vi "Get Value.vi"(8 "error in (no error)":errorcluster, 11 "SingleA in":refnum<class "SingleA.lvclass">) -> (0 "error out":errorcluster, 2 "value":dbl, 3 "SingleA out":refnum<class "SingleA.lvclass">)   [LabVIEW 2020, in "SingleA.lvclass"]
uses:
  SingleA.lvclass
  D:/03 GitHub/LabVIEW-Singleton/Singleton/Singleton.lvclass
  Singleton/Singleton.lvclass/Singleton.ctl
  SingleA.lvclass/SingleA.ctl
  Singleton/Singleton.lvclass
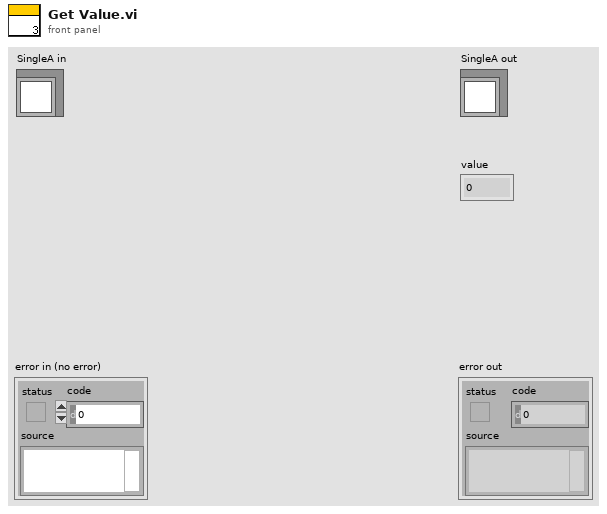
[diagram p1: front panel]
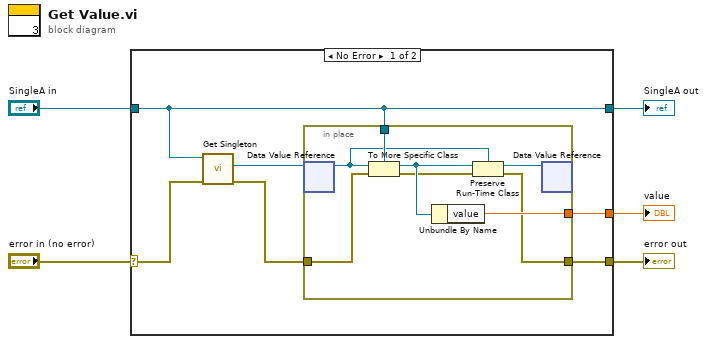
[diagram p0: block diagram]
diagram:
  n1 = case shown="No Error" "error in (no error)" {
    selector: "error in (no error)" -> [w8 w21]
    tunnel: [w7 w21] -> w4
    tunnel: [w10 w20] -> w2
    tunnel: "SingleA in" -> [w10 w20]
    tunnel: [w9 _] -> w1
    frame No Error {
      n2 = call "Get Singleton.vi"("error in (no error)"=w8, "Singleton in"=w10) -> ("error out"=w6:errorcluster, "singleton"=w11:refnum<data-value>)  [unwired: 7 in, 1 out]
      n3 = in-place {
        in-place-border: w10 -> [w19]
        in-place-border: [w15] -> w9
        in-place-border: w6 -> [w14]
        in-place-border: [w12] -> w7
        n4 = in-place-dvr #1(w11) -> (w18:refnum<class>)  [unwired: 1 out]
        n5 = To More Specific Class(target class=w19, reference=w18, error in=w14) -> (specific class reference=w16:refnum<class "SingleA.lvclass">, error out=w13:errorcluster)
        n6 = Unbundle By Name(w16) -> ("value"=w15:dbl)
        n7 = Preserve Run-Time Class(object in=w16, error in=w13, 2:w18) -> (object out=w17:refnum<class>, error out=w12:errorcluster)
        n8 = in-place-dvr #1(w17) -> ()  [unwired: 2 out]
      }
    }
    frame Error {
    }
  }
  "error out" <- w4
  "SingleA out" <- w2
  "value" <- w1
